vi "Add Pulse Recorders.vi"(8 "error in (no error)":errorcluster, 9 "Auto launch":bool=TRUE, 10 "Module type":T1, 11 "Monitor-Pulse in":refnum<class "Monitor-Pulse.lvclass">) -> (0 "error out":errorcluster, 1 "Actor names out":string[](array[string]), 2 "Recorders out":refnum<class "Pulse Recorder.lvclass">[](array[class]), 3 "Monitor-Pulse out":refnum<class "Monitor-Pulse.lvclass">)   [LabVIEW 2016, in "Monitor-Pulse.lvclass"]
uses:
  Monitor-Pulse.lvclass
  Pulse Recorders/Pulse Recorder/Pulse Recorder.lvclass
  C:/Github/LabActor/Template Module/Template Module.lvclass
  C:/Github/LabActor/Worker/Worker.lvclass
  Module Types.ctl
  NHMFL_Core/Libraries/Instruments/Instrument Driver/Instrument Driver.lvclass/Instrument Driver.ctl
  Recorders/RP I-V/RP I-V.lvclass
  C:/Github/LabActor/Pulse Recorders/Pulse Recorder/Pulse Recorder.lvclass
  Template Module/Template Module.lvclass/Template Module.ctl
  NHMFL_Core/Libraries/Instruments/Instrument Driver/Read Type ID.vi
  Template Module/Write Name.vi
  NHMFL_Core/Libraries/Red Pitaya/Red Pitaya Digitizer/Red Pitaya Digitizer.lvclass
  C:/Github/NHMFL_Core/Libraries/Instruments/Pulse Driver/Pulse Driver.lvclass
  NHMFL_Core/Libraries/Instruments/Pulse Driver/Pulse Driver.lvclass
  C:/Github/NHMFL_Core/Libraries/Instruments/Instrument Driver/Instrument Driver.lvclass
  Pulse Recorders/Pulse Recorder/Write Pulse driver.vi
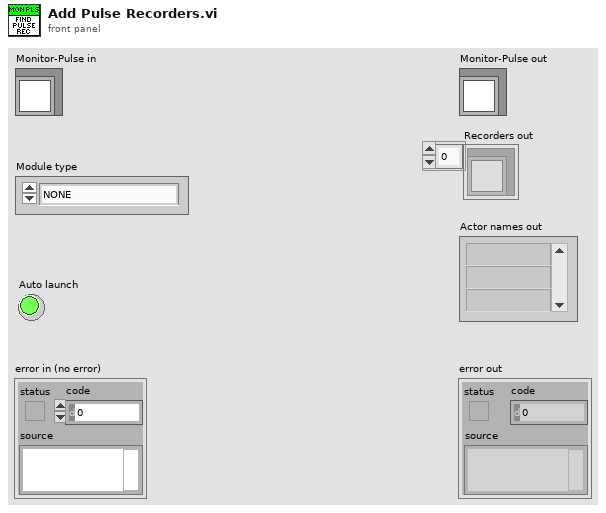
[diagram p1: front panel]
types:
  T1 = typedef "Module Types.ctl" = enum16{"NONE", "NI-DAQmx", "NI-Scope", "Red Pitaya Digitizer", "GaGe", "VISA Device", "Red Pitaya Lockin", "Monitor Controller", "Pulse Controller", "Integrate Pulse", "Lockin Processor", "File converter", "NHMFL Synthesizer", "Micron Hyperion", "Spectrum Recorder", "Line Detector", "TCP Communications", "Elastic Moduli"}
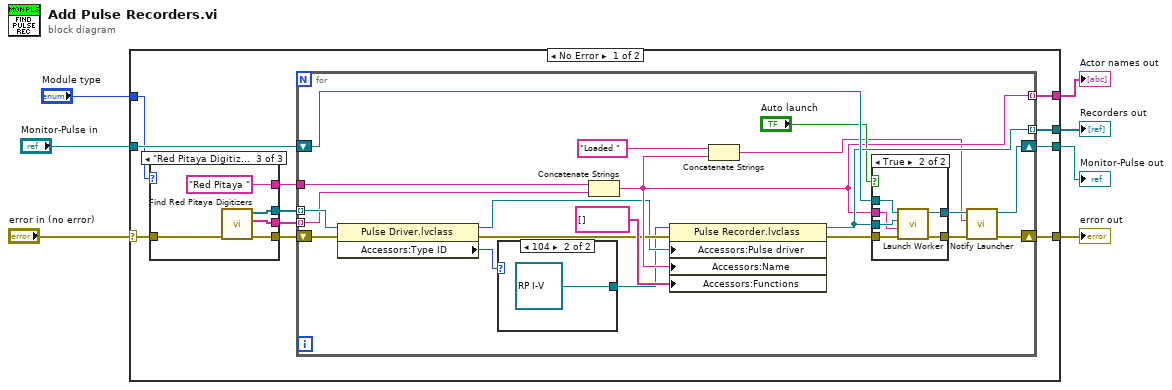
[diagram p0: block diagram]
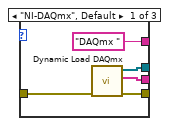
[diagram p2: hidden frame]
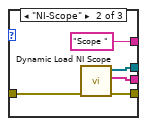
[diagram p3: hidden frame]
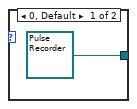
[diagram p4: hidden frame]
diagram:
  n1 = case shown="No Error" "error in (no error)" {
    selector: "error in (no error)" -> [w18 w65]
    tunnel: [w14 w65] -> w6
    tunnel: [w10 w64] -> w4
    tunnel: "Monitor-Pulse in" -> [w11 w64]
    tunnel: [w13 _] -> w3
    tunnel: [w12 _] -> w2
    tunnel: "Module type" -> [w9 _]
    frame No Error {
      n2 = case shown="\"Red Pitaya Digitizer\"" w9 {
        tunnel: w18 -> [w23 w28 w33]
        tunnel: [w22 w25 w30] -> w17
        tunnel: [w21 w27 w29] -> w16
        tunnel: [w20 w26 w32] -> w15
        tunnel: ["DAQmx " "Scope " "Red Pitaya "] -> w8
        frame "NI-DAQmx", Default {
          n3 = call "Dynamic Load DAQmx.vi"("Error In"=w23) -> ("Error Out"=w21:errorcluster, "Device names"=w20:string[], "Digitizers out"=w22:refnum<class "Pulse Driver.lvclass">[])  [unwired: 8 in]
        }
        frame "NI-Scope" {
          n4 = call "Dynamic Load NI Scope.vi"("Error In"=w28) -> ("Error Out"=w27:errorcluster, "Device names"=w26:string[], "Digitizers out"=w25:refnum<class "Pulse Driver.lvclass">[])  [unwired: 8 in]
        }
        frame "Red Pitaya Digitizer" {
          n5 = call "Find Red Pitaya Digitizers.vi"("Error In"=w33) -> ("Error Out"=w29:errorcluster, "Device names"=w32:string[], "Digitizers out"=w30:refnum<class "Red Pitaya Digitizer.lvclass">[])  [unwired: 7 in, 1 out]
        }
      }
      n6 = for {
        tunnel: w17 -> [w38] mode=indexing
        shift-right: [w44] -> w14
        shift-left: w16 -> [w53]
        tunnel: w15 -> [w34] mode=indexing
        tunnel: [w51] -> w13 mode=indexing
        tunnel: [w42] -> w12 mode=indexing
        shift-right: [w46] -> w10
        shift-left: w11 -> [w52]
        tunnel: w8 -> [w48]
        n7 = property class="Pulse Driver.lvclass"(reference=w38, error in=w53) -> (reference out=w37:refnum<class "Pulse Driver.lvclass">, error out=w39:errorcluster, "Accessors:Type ID"=w36:i32)
        n8 = case shown="104" w36 {
          tunnel: [refnum<class "Pulse Recorder.lvclass"> refnum ("Pulse Recorder.lvclass") refnum<class "RP I-V.lvclass"> refnum ("RP I-V.lvclass")] -> w35
          frame 0, Default {
          }
          frame 104 {
          }
        }
        n9 = Concatenate Strings(w48, w34) -> (w42:string)
        n10 = property class="Pulse Recorder.lvclass"(reference=w35, error in=w39, "Accessors:Pulse driver"=w37, "Accessors:Name"=w42, "Accessors:Functions"=string[] [] ("Functions")) -> (reference out=w51:refnum<class "Pulse Recorder.lvclass">, error out=w50:errorcluster)
        n11 = Concatenate Strings("Loaded " ("string"), w42) -> (w41:string)
        n12 = case shown="True" "Auto launch" {
          tunnel: w52 -> [w57 w63]
          tunnel: w51 -> [_ w62]
          tunnel: [w57 w61] -> w47
          tunnel: w50 -> [w56 w60]
          tunnel: [w56 w59] -> w45
          tunnel: w42 -> [_ w58]
          frame False {
          }
          frame True {
            n13 = call-dynamic "Launch Worker.vi"("error in (no error)"=w60, "Name"=w58, "Subordinate Object"=w62, "Application Controller in"=w63) -> ("error out"=w59:errorcluster, "Application Controller out"=w61:refnum<class "Monitor-Pulse.lvclass">)  [unwired: 5 in, 1 out]
          }
        }
        n14 = call-dynamic "Notify Launcher.vi"("error in (no error)"=w45, "Notification"=w41, "Application Controller in"=w47) -> ("error out"=w44:errorcluster, "Application Controller out"=w46:refnum<class "Monitor-Pulse.lvclass">)  [unwired: 7 in]
      }
    }
    frame Error {
    }
  }
  "error out" <- w6
  "Monitor-Pulse out" <- w4
  "Recorders out" <- w3
  "Actor names out" <- w2
